vi "waveformAttributes.vi"() -> ()   [LabVIEW 2014]
uses:
  <vilib>/measure/NI_MABase.lvlib
panel:
  in  "Poisson Mean":dbl(knob)=10.0 scale=0.0..50.0
  in  "Poisson Sampling Settings":T1={"Sampling Frequency"=1000.0, "Number of Samples"=1000.0} {"Number of Samples" scale=0.0..1000.0; "Sampling Frequency" scale=0.0..5000.0}
  in  "Channel Units":string="FakeVolts"
  in  "Channel Name":string="Sine Signal"
  out "Waveform Graph":waveform(dbl)(graph)
  out "Waveform Attributes":cluster{string, variant}[](array[cluster])
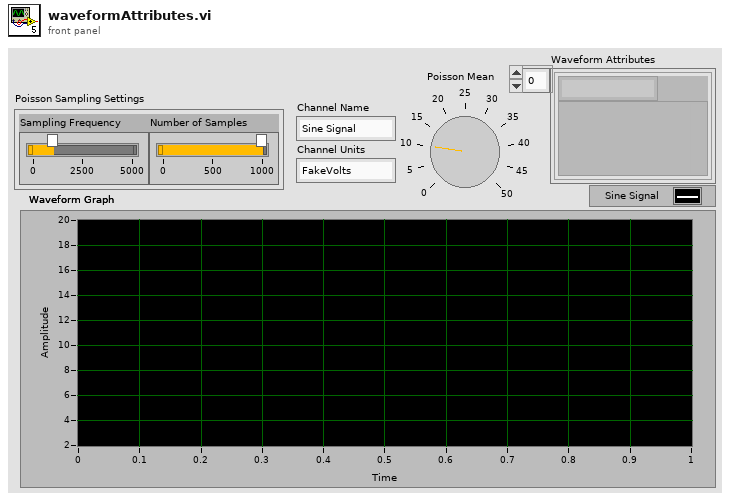
[diagram p1: front panel]
types:
  T1 = cluster{"Sampling Frequency":dbl, "Number of Samples":dbl}
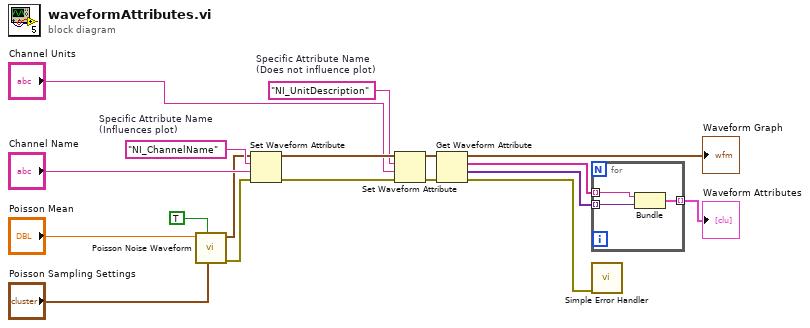
[diagram p0: block diagram]
diagram:
  w9 = "NI_UnitDescription"  # Specific Attribute Name (Does not influence plot)
  w11 = "NI_ChannelName"  # Specific Attribute Name (Influences plot)
  n1 = call <vilib>:"Poisson Noise Waveform.vi"("sampling info"="Poisson Sampling Settings", "reset signal"=TRUE, "mean"="Poisson Mean") -> ("error out"=w5:errorcluster, "signal out"=w7:waveform(dbl))  [unwired: 7 in]
  n2 = Set Waveform Attribute(4:w5, 5:"Channel Name", 6:w11, 7:w7) -> (0:w4:errorcluster, 3:w12:waveform(dbl))  [unwired: 1 out]
  n3 = Set Waveform Attribute(4:w4, 5:"Channel Units", 6:w9, 7:w12) -> (0:w3:errorcluster, 3:w6:waveform(dbl))  [unwired: 1 out]
  n4 = Get Waveform Attribute(4:w3, 7:w6) -> (0:w2:errorcluster, 1:w17:variant[], 2:w18:string[], 3:→"Waveform Graph":waveform(dbl))  [unwired: 2 in]
  n5 = for {
    tunnel: w18 -> [w21] mode=indexing
    tunnel: w17 -> [w20] mode=indexing
    tunnel: [w19] -> w16 mode=indexing
    n6 = Bundle(w21, w20) -> (w19:cluster{string, variant})  [unwired: 1 in]
  }
  "Waveform Attributes" <- w16
  n7 = call <vilib>:"Simple Error Handler.vi"("error in (no error)"=w2) -> ()  [unwired: 4 in, 5 out]
